vi "Configure Acquisition.vi"(8 "error in":errorcluster, 11 "DS1054 Base CFG in":refnum<class "DS1054 Base CFG.lvclass">) -> (0 "error out":errorcluster, 3 "DS1054 Base CFG out":refnum<class "DS1054 Base CFG.lvclass">)   [LabVIEW 2023, in "RIGOL DS1054Z.lvlib" / "DS1054 Base CFG.lvclass"]
uses:
  DS1054 Base CFG.lvclass
  Scope/Scope VISA/Configuration/Scope VISA CFG.lvclass/Scope VISA CFG.ctl
  Configuration Base/Configuration Base.lvclass/Configuration Base.ctl
  41a4d43c-b518-44d9-b428-0b31f9eb17dc.vi
  7e90698c-744c-41e6-ab3b-f781ce1178e6.vi
  af8d73a0-154d-4613-b104-ac55ae7eb0f7.vi
  <vilib>/JDP Science/JSONtext/Next JSON Value.vi
  <vilib>/JDP Science/JSONtext/String Subset.vi
  <vilib>/JDP Science/JSONtext/Parsing/Advance past next JSON Value (inlined COPY).vi
  <vilib>/JDP Science/JSONtext/Parsing/Advance past whitespace.vi
  <vilib>/JDP Science/JSONtext/Parsing/Advance past String.vi
  <vilib>/JDP Science/JSONtext/Parsing/Advance past Number.vi
  <vilib>/JDP Science/JSONtext/Parsing/Advance past Line Ending.vi
  <vilib>/JDP Science/JSONtext/Parsing/Parse Full Path or Item Name.vi
  <vilib>/JDP Science/JSONtext/Parsing/Advance past Array.vi
  <vilib>/JDP Science/JSONtext/Parsing/Advance past Object.vi
  <vilib>/JDP Science/JSONtext/support/Error Cluster From Code.vi
  <vilib>/JDP Science/JSONtext/Offset/Find Item Locations by Path.vi
  <vilib>/JDP Science/JSONtext/JSON text to Variant.vi
  <vilib>/Utility/error.llb/Error Cluster From Error Code.vi
  <vilib>/JDP Science/JSONtext/LVClass Serializer/JSONtext LVClass Serializer.lvclass
  <vilib>/ErrorRing/Error Ring.xnode
  Configuration Base/Configuration Base.lvclass
  <vilib>/JDP Science/JSONtext/JSONtext.lvlib
  Scope/Scope VISA/Configuration/Scope VISA CFG.lvclass
  <instrlib>/RIGOL-DS1054Z-LabVIEW/RIGOL DS1054Z Driver.lvlib
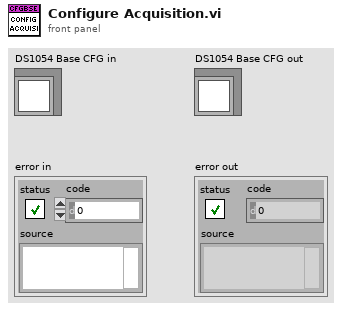
[diagram p1: front panel]
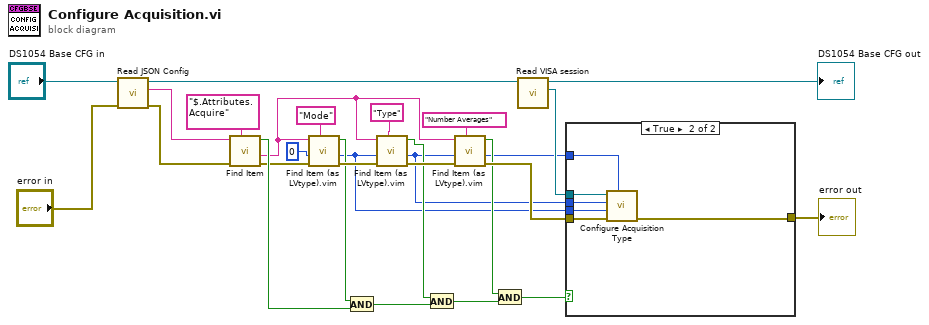
[diagram p0: block diagram]
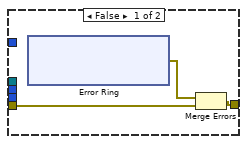
[diagram p2: hidden frame]
diagram:
  n1 = call "Read JSON Config.vi"("error in"="error in", "object in"="DS1054 Base CFG in") -> ("error out"=w24:errorcluster, "<JSON>Config"=w25:string, "object out"=w26:refnum<class "DS1054 Base CFG.lvclass">)  [unwired: 7 in]
  n2 = call <vilib>:"Find Item.vi"("$Path or Item Name"="$.Attributes.Acquire", "error in (no error)"=w24, "JSON"=w25) -> ("error out"=w21:errorcluster, "<JSON>"=w11:string, "Found"=w23:bool)  [unwired: 5 in, 1 out]
  n3 = call "Find Item (as LVtype).vim"("$Path or Item Name"="Mode", "error in (no error)"=w21, "Data Type and Default Value"=0, "JSON"=w11) -> ("error out"=w15:errorcluster, "Data"=w4:i32, "Found"=w8:bool)  [unwired: 4 in, 1 out]
  n4 = And(x=w8, y=w23) -> (x .and. y?=w10:bool)
  n5 = call "Find Item (as LVtype).vim"("$Path or Item Name"="Type", "error in (no error)"=w15, "Data Type and Default Value"=w4, "JSON"=w11) -> ("error out"=w14:errorcluster, "Data"=w5:i32, "Found"=w9:bool)  [unwired: 4 in, 1 out]
  n6 = And(x=w9, y=w10) -> (x .and. y?=w6:bool)
  n7 = call "Find Item (as LVtype).vim"("$Path or Item Name"="Number Averages", "error in (no error)"=w14, "Data Type and Default Value"=w5, "JSON"=w11) -> ("error out"=w13:errorcluster, "Data"=w3:i32, "Found"=w7:bool)  [unwired: 4 in, 1 out]
  n8 = And(x=w7, y=w6) -> (x .and. y?=w2:bool)
  n9 = call "Read VISA session.vi"("Scope VISA CFG in"=w26) -> ("VISA session"=w18:refnum<visa-resource-name>, "Scope VISA CFG out"=→"DS1054 Base CFG out":refnum<class "DS1054 Base CFG.lvclass">)  [unwired: 8 in, 1 out]
  n10 = case shown="True" w2 {
    tunnel: w18 -> [_ w42]
    tunnel: w13 -> [w30 w41]
    tunnel: w5 -> [_ w40]
    tunnel: w4 -> [_ w39]
    tunnel: w3 -> [_ w38]
    tunnel: [w29 w37] -> w1
    frame False {
      n11 = xnode "Error Ring"() -> ("error out"=w31:errorcluster)
      n12 = Merge Errors(w31, w30) -> (w29:errorcluster)
    }
    frame True {
      n13 = call <instrlib>:"Configure Acquisition Type.vi"("Number Of Averages (8)"=w38, "error in (no error)"=w41, "Acquisition Mode (0: Real time)"=w39, "Acquisition Type (0: Normal)"=w40, "VISA resource name"=w42) -> ("error out"=w37:errorcluster)  [unwired: 5 in, 1 out]
    }
  }
  "error out" <- w1
